vi "Username Dialog.vi"(8 "Error In":errorcluster, 11 "Username In":string) -> (0 "Error Out":errorcluster, 3 "Username Out":string)   [LabVIEW 2017, in "Tests.lvlib"]
uses:
  Tests.lvlib
panel:
  in  "Cancel":bool
  in  "OK":bool
  in  "Username":string
  # "SSH TEST SERVER USERNAME"
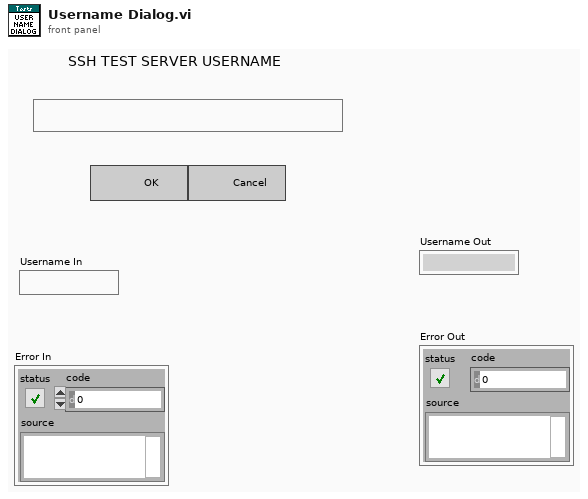
[diagram p1: front panel]
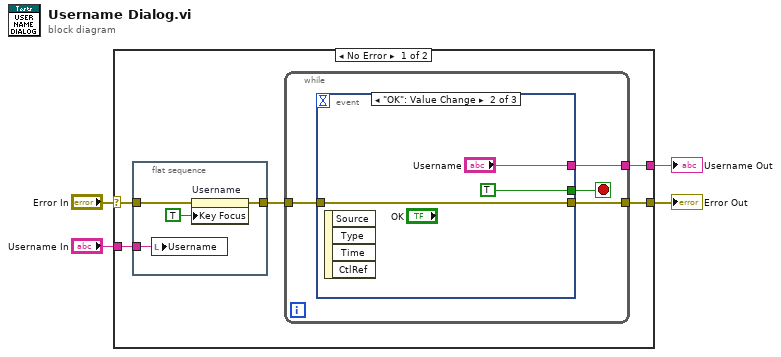
[diagram p0: block diagram]
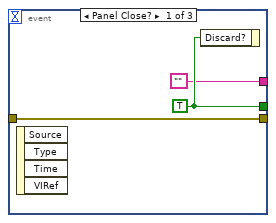
[diagram p2: hidden frame]
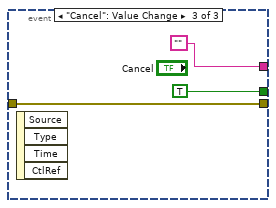
[diagram p3: hidden frame]
diagram:
  n1 = case shown="No Error" "Error In" {
    selector: "Error In" -> [w7 w27]
    tunnel: [w9 w27] -> w3
    tunnel: [w5 _] -> w2
    tunnel: "Username In" -> [w8 _]
    frame No Error {
      n2 = flat-sequence {
        tunnel: w8 -> [w13]
        tunnel: w7 -> [w12]
        tunnel: [w11] -> w6
        frame #0 {
          n3 = local write "Username"(w13) -> ()
          n4 = property on="Username" class="Str"(error in=w12, "Key Focus"=TRUE) -> (error out=w11:errorcluster)  [unwired: 1 in, 1 out]
        }
      }
      n5 = while {
        tunnel: w6 -> [w16]
        tunnel: [w15] -> w9
        tunnel: [w14] -> w5
        stop <- w17 stop-if-true
        n6 = event shown="[1] \"OK\": Value Change" {
          selector: _ -> [_ _ _]
          dyn-events: _ -> [_ _ _]
          timeout: _ -> [_ _ _]
          tunnel: [w20 TRUE TRUE] -> w17
          tunnel: w16 -> [w19 w23 w26]
          tunnel: [w19 w23 w26] -> w15
          tunnel: ["" "Username" ""] -> w14
          event Panel Close? {
            w20 = TRUE
            n7 = event-data() -> ()  [unwired: 1 in, 4 out]
            n8 = event-data("Discard?"=w20) -> ()  [unwired: 1 in, 1 out]
          }
          event "OK": Value Change {
            n9 = event-data() -> ()  [unwired: 1 in, 4 out]
          }
          event "Cancel": Value Change {
            n10 = event-data() -> ()  [unwired: 1 in, 4 out]
          }
        }
      }
    }
    frame Error {
    }
  }
  "Error Out" <- w3
  "Username Out" <- w2
